vi "Sensor handling full_ext.vi"(0 "PV":dbl step=0.009999999776482582, 1 "SOURCE":u32=1 max=2 step=1, 2 "SOURCE_ALLOW":bool, 3 "PV2":dbl step=0.009999999776482582, 4 "control":T2={"GAIN"=1.0, "OFFSET"=0.0, "TIME_CONST"=100.0, "MINOFFSET"=2.0, "PVMIN"=0.0, "MINACC"=0.0, "LL"=1.0, "L"=2.0, "H"=8.0, "HH"=9.0, "MAXACC"=9.5, "PVMAX"=10.0, "MAXOFFSET"=2.0, "D"=0.5, "input_register_min"=0.0, "input_register_max"=100.0, "input_pv_min"=0.0, "input_pv_max"=100.0, "VMAX"=0.0, "TOUT"=1.0, "APERTURE"=0.0} {"input_pv_max" min=-100000.0 max=100000.0 step=0.0010000000474974513; "input_pv_min" min=-100000.0 max=100000.0 step=0.0010000000474974513; "input_register_max" min=-100000.0 max=100000.0 step=0.0010000000474974513; "input_register_min" min=-100000.0 max=100000.0 step=0.0010000000474974513; "APERTURE" min=-100000.0 max=100000.0 step=0.0010000000474974513; "TOUT" min=0.0 max=100000.0 step=1.0; "D" min=-100000.0 max=100000.0 step=0.0010000000474974513; "MAXOFFSET" min=0.0 max=50.0 step=0.0010000000474974513; "PVMAX" min=-100000.0 max=100000.0 step=0.0010000000474974513; "MAXACC" min=-100000.0 max=100000.0 step=0.0010000000474974513; "HH" min=-100000.0 max=100000.0 step=0.0010000000474974513; "H" min=-100000.0 max=100000.0 step=0.0010000000474974513; "L" min=-100000.0 max=100000.0 step=0.0010000000474974513; "LL" min=-100000.0 max=100000.0 step=0.0010000000474974513; "MINACC" min=-100000.0 max=100000.0 step=0.0010000000474974513; "PVMIN" min=-100000.0 max=100000.0 step=0.0010000000474974513; "MINOFFSET" min=0.0 max=50.0 step=0.0010000000474974513; "TIME_CONST" min=1.0 max=100000.0 step=1.0; "OFFSET" min=-100000.0 max=100000.0 step=0.0010000000474974513; "GAIN" min=0.0010000000474974513 max=1000.0 step=0.0010000000474974513}, 6 "initialise":bool, 7 "Sensor handling full reg old":T1, 8 "connect":bool) -> (13 "Sensor handling full reg":T1, 14 "PVOUT":dbl format="%#_3g", 15 "SOURCEOUT":u32=1 max=2 step=1, 16 "STATE":T3, 17 "block":u32 format="%09b", 19 "ALRSTATE":errorcluster)   [LabVIEW 2019, in "Inputs.lvlib"]
uses:
  Inputs.lvlib
  Ctl/Parameter State.ctl
  Ctl/Sensor state.ctl
  Ctl/Sensor alarm.ctl
  Sensor_limit_Hd.vi
  Sensor_limit_Ld.vi
  Sensor_limit_H.vi
  Sensor_limit_L.vi
  Userlib.lvlib
  Trigers/Triggers.lvlib
panel:
  in  "UNIT":string
  in  "SENSOR":string
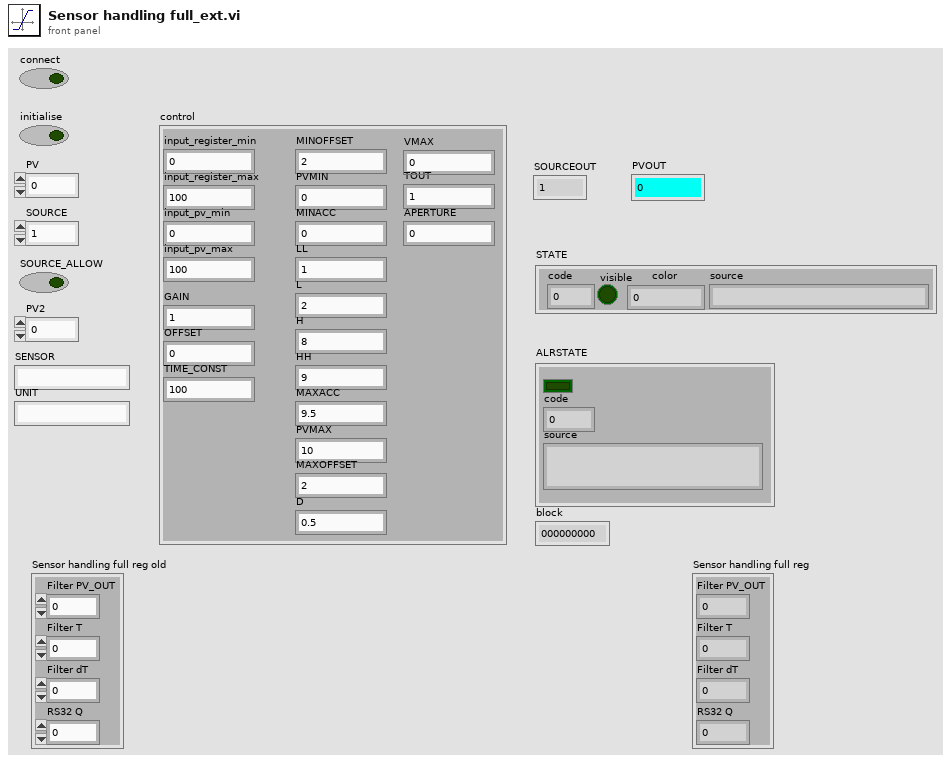
[diagram p1: front panel]
types:
  T1 = cluster{"Filter PV_OUT":dbl, "Filter T":dbl, "Filter dT":dbl, "RS32 Q":u32}
  T2 = cluster{"GAIN":dbl, "OFFSET":dbl, "TIME_CONST":dbl, "MINOFFSET":dbl, "PVMIN":dbl, "MINACC":dbl, "LL":dbl, "L":dbl, "H":dbl, "HH":dbl, "MAXACC":dbl, "PVMAX":dbl, "MAXOFFSET":dbl, "D":dbl, "input_register_min":dbl, "input_register_max":dbl, "input_pv_min":dbl, "input_pv_max":dbl, "VMAX":dbl, "TOUT":dbl, "APERTURE":dbl}
  T3 = typedef "Inputs.lvlib/Parameter State.ctl" = cluster{"code":i32, "visible":bool, "color":u32, "source":string}
  T4 = typedef "Inputs.lvlib/Sensor state.ctl" = cluster{"source":string, "color":u32, "visible":bool}[]
  T5 = typedef "Inputs.lvlib/Sensor alarm.ctl" = cluster{"source":string, "color":u32, "visible":bool}[]
  T6 = cluster{"source":string, "color":u32, "visible":bool}
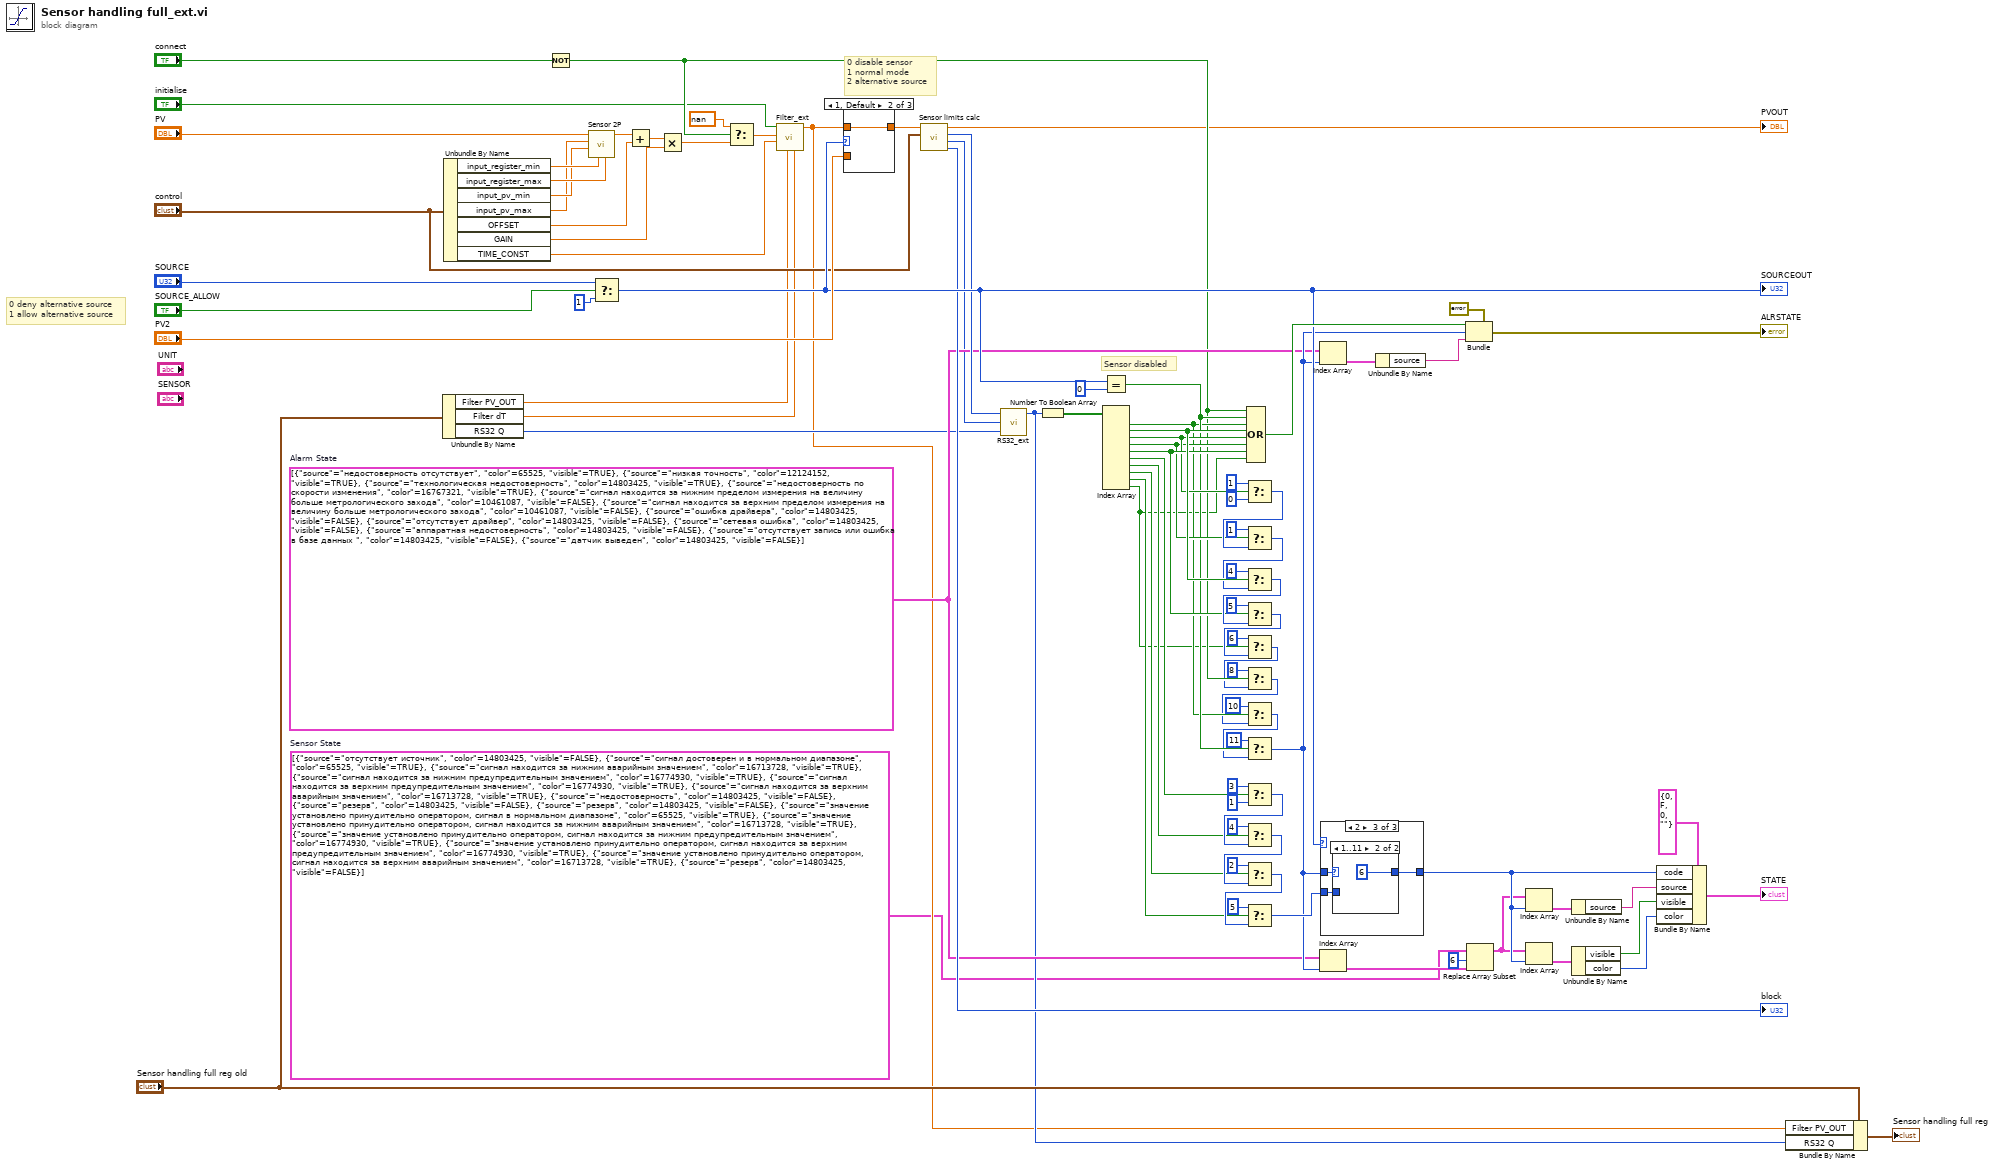
[diagram p0: block diagram]
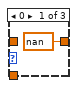
[diagram p2: hidden frame]
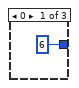
[diagram p4: hidden frame]
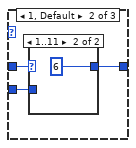
[diagram p5: hidden frame]
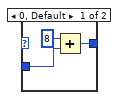
[diagram p7: hidden frame]
diagram:
  w1 = T4 [{"source"="отсутствует источник", "color"=14803425, "visible"=FALSE}, {"source"="сигнал достоверен и в нормальном диапазоне", "color"=65525, "visible"=TRUE}, {"source"="сигнал находится за нижним аварийным значением", "color"=16713728, "visible"=TRUE}, {"source"="сигнал находится за нижним предупредительным значением", "color"=16774930, "visible"=TRUE}, {"source"="сигнал находится за верхним предупредительным значением", "color"=16774930, "visible"=TRUE}, {"source"="сигнал находится за верхним аварийным значением", "color"=16713728, "visible"=TRUE}, {"source"="недостоверность", "color"=14803425, "visible"=FALSE}, {"source"="резерв", "color"=14803425, "visible"=FALSE}, {"source"="резерв", "color"=14803425, "visible"=FALSE}, {"source"="значение установлено принудительно оператором, сигнал в нормальном диапазоне", "color"=65525, "visible"=TRUE}, {"source"="значение установлено принудительно оператором, сигнал находится за нижним аварийным значением", "color"=16713728, "visible"=TRUE}, {"source"="значение установлено принудительно оператором, сигнал находится за нижним предупредительным значением", "color"=16774930, "visible"=TRUE}, {"source"="значение установлено принудительно оператором, сигнал находится за верхним предупредительным значением", "color"=16774930, "visible"=TRUE}, {"source"="значение установлено принудительно оператором, сигнал находится за верхним аварийным значением", "color"=16713728, "visible"=TRUE}, {"source"="резерв", "color"=14803425, "visible"=FALSE}]  # Sensor State
  w25 = T5 [{"source"="недостоверность отсутствует", "color"=65525, "visible"=TRUE}, {"source"="низкая точность", "color"=12124152, "visible"=TRUE}, {"source"="технологическая недостоверность", "color"=14803425, "visible"=TRUE}, {"source"="недостоверность по скорости изменения", "color"=16767321, "visible"=TRUE}, {"source"="сигнал находится за нижним пределом измерения на величину больше метрологического захода", "color"=10461087, "visible"=FALSE}, {"source"="сигнал находится за верхним пределом измерения на величину больше метрологического захода", "color"=10461087, "visible"=FALSE}, {"source"="ошибка драйвера", "color"=14803425, "visible"=FALSE}, {"source"="отсутствует драйвер", "color"=14803425, "visible"=FALSE}, {"source"="сетевая ошибка", "color"=14803425, "visible"=FALSE}, {"source"="аппаратная недостоверность", "color"=14803425, "visible"=FALSE}, {"source"="отсутствует запись или ошибка в базе данных ", "color"=14803425, "visible"=FALSE}, {"source"="датчик выведен", "color"=14803425, "visible"=FALSE}]  # Alarm State
  # "Sensor disabled"
  # "0 disable sensor\n1 normal mode\n2 alternative source"
  # "0 deny alternative source\n1 allow alternative source"
  n1 = Unbundle By Name("Sensor handling full reg old") -> ("Filter PV_OUT"=w20:dbl, "Filter dT"=w19:dbl, "RS32 Q"=w18:u32)
  n2 = Unbundle By Name("control") -> ("input_register_min"=w31:dbl, "input_register_max"=w30:dbl, "input_pv_min"=w29:dbl, "input_pv_max"=w28:dbl, "OFFSET"=w69:dbl, "GAIN"=w68:dbl, "TIME_CONST"=w21:dbl)
  n3 = Not(x="connect") -> (.not. x?=w14:bool)
  n4 = call "Sensor 2P.vi"("Xmax"=w30, "Xmin"=w31, "Ymin"=w29, "Ymax"=w28, "X"="PV") -> ("Y"=w33:dbl)  [unwired: 6 in]
  n5 = Select(t="SOURCE", s="SOURCE_ALLOW", f=u32 1) -> (s? t:f=w64:u32)
  "SOURCEOUT" <- w64
  n6 = Add(x=w33, y=w69) -> (x+y=w91:dbl)
  n7 = Multiply(x=w91, y=w68) -> (x*y=w16:dbl)
  n8 = Select(t=nan, s=w14, f=w16) -> (s? t:f=w15:dbl)
  n9 = call "Filter_ext.vi"("dT"=w19, "PV_OUT old"=w20, "time_const ms"=w21, "PV"=w15, "Initialise"="initialise") -> ("PV_OUT"=w2:dbl)  [unwired: 6 in]
  n10 = case shown="1, Default" w64 {
    tunnel: w2 -> [_ w93 _]
    tunnel: [nan w93 w94] -> w50
    tunnel: "PV2" -> [_ _ w94]
    frame 0 {
    }
    frame 1, Default {
    }
    frame 2 {
    }
  }
  n11 = call "Sensor limits calc.vi"("control"="control", "PV"=w50) -> ("block"=→"block":u32, "Off"=w23:u32, "On"=w49:u32, "PVOUT"=→"PVOUT":dbl)  [unwired: 2 in]
  n12 = call "RS32_ext.vi"("Q old"=w18, "R"=w23, "S"=w49) -> ("Q"=w3:u32)  [unwired: 1 in, 1 out]
  n13 = Number To Boolean Array(number=w3) -> (Boolean array=w71:bool[])
  n14 = Equal?(x=w64, y=u32 0) -> (x = y?=w53:bool)
  n15 = Index Array(array=w71) -> (element #1=w51:bool, element #2=w70:bool, element #3=w55:bool, element #4=w54:bool, element #5=w59:bool, element #6=w60:bool, element #7=w61:bool, element #8=w62:bool, element #9=w63:bool, element #10=w8:bool)  [unwired: 10 in]
  n16 = Compound Arithmetic op=OR ("status")(w14, w53, w51, w70, w55, w54, w59, w8) -> (w76:bool)
  n17 = Select ("code")(t=1, s=w55, f=0) -> (s? t:f=w57:i32)
  n18 = Select ("code")(t=1, s=w54, f=w57) -> (s? t:f=w56:i32)
  n19 = Select ("code")(t=4, s=w70, f=w56) -> (s? t:f=w85:i32)
  n20 = Select ("code")(t=5, s=w59, f=w85) -> (s? t:f=w10:i32)
  n21 = Select ("code")(t=6, s=w8, f=w10) -> (s? t:f=w9:i32)
  n22 = Select ("code")(t=8, s=w14, f=w9) -> (s? t:f=w34:i32)
  n23 = Select ("code")(t=10, s=w51, f=w34) -> (s? t:f=w40:i32)
  n24 = Select ("code")(t=11, s=w53, f=w40) -> (s? t:f=w46:i32)
  n25 = Select ("code")(t=3 ("code"), s=w60, f=1 ("code")) -> (s? t:f=w80:i32)
  n26 = Select ("code")(t=4 ("code"), s=w61, f=w80) -> (s? t:f=w79:i32)
  n27 = Select ("code")(t=2 ("code"), s=w62, f=w79) -> (s? t:f=w77:i32)
  n28 = Select ("code")(t=5 ("code"), s=w63, f=w77) -> (s? t:f=w72:i32)
  n29 = Index Array(array=w25, index=w46) -> (element=w44:T6)
  n30 = Index Array(array=w25, index=w46) -> (element=w43:T6)
  n31 = case "code" shown="2" w64 {
    tunnel: w46 -> [_ w98 w103]
    tunnel: w72 -> [_ w97 w102]
    tunnel: [6 ("code") w96 w101] -> w38
    frame 0 {
    }
    frame 1, Default {
      n32 = case "code" shown="1..11" w98 {
        tunnel: [w99 6 ("code")] -> w96
        tunnel: w97 -> [w99 _]
        frame 0, Default {
        }
        frame 1..11 {
        }
      }
    }
    frame 2 {
      n33 = case "code" shown="1..11" w103 {
        tunnel: [w105 6 ("code")] -> w101
        tunnel: w102 -> [w106 _]
        frame 0, Default {
          n34 = Add ("code")(x=8 ("code"), y=w106) -> (x+y=w105:i32)
        }
        frame 1..11 {
        }
      }
    }
  }
  n35 = Unbundle By Name(w44) -> ("source"=w45:string)
  n36 = Bundle(cluster=cluster{bool, i32, "source":string} {FALSE, 0, "source"=""}, w76, w46, "source"=w45) -> (→"ALRSTATE":cluster{bool, i32, "source":string})
  n37 = Replace Array Subset(array=w1, new element=w43, index=6) -> (w7:T4)
  n38 = Index Array(array=w7, index=w38) -> (element=w39:T6)
  n39 = Index Array(array=w7, index=w38) -> (element=w41:T6)
  n40 = Unbundle By Name(w39) -> ("source"=w42:string)
  n41 = Unbundle By Name(w41) -> ("visible"=w37:bool, "color"=w27:u32)
  n42 = Bundle By Name(cluster=T3 {"code"=0, "visible"=FALSE, "color"=0, "source"=""} ("STATE"), "code"=w38, "source"=w42, "visible"=w37, "color"=w27) -> (→"STATE":T3)
  n43 = Bundle By Name(cluster="Sensor handling full reg old", "Filter PV_OUT"=w2, "RS32 Q"=w3) -> (→"Sensor handling full reg":T1)
